vi "Build Description String.vi"(8 "error in (no error)":errorcluster, 11 "Keyboard Action in":refnum<class "Keyboard Action.lvclass">) -> (0 "error out":errorcluster, 1 "Description":string, 2 "Subtype String":string, 3 "Keyboard Action out":refnum<class "Keyboard Action.lvclass">)   [LabVIEW 2020, in "MacroAssert.lvlib" / "Keyboard Action.lvclass"]
doc: "Builds a string to describe what <B>Step</B> does."
uses:
  Keyboard Action.lvclass
  Keyboard Action.lvclass/Keyboard Action.ctl
  MacroAssert.lvlib
panel:
  in  "Virtual Key":u8(ring)=65
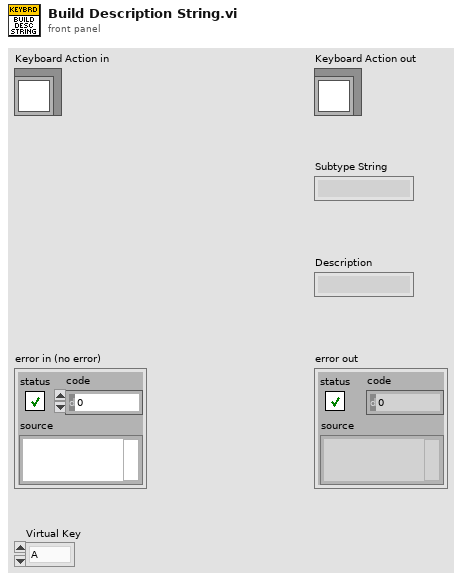
[diagram p1: front panel]
types:
  T1 = typedef "MacroAssert.lvlib/Keyboard Action.lvclass/Keyboard Action Type.ctl" = enum16{"Key Press", "Key Sequence", "Key Down", "Key Up"}
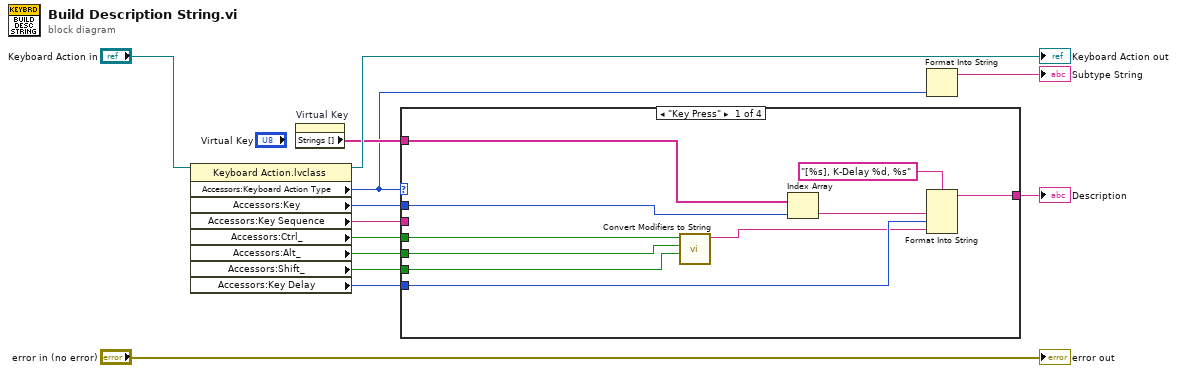
[diagram p0: block diagram]
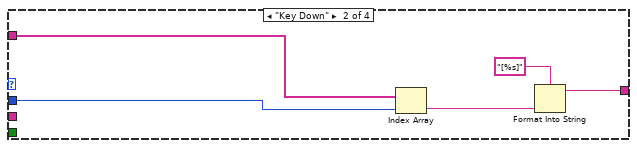
[diagram p2: hidden frame]
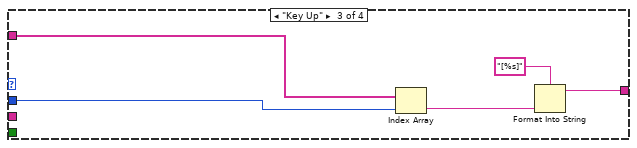
[diagram p3: hidden frame]
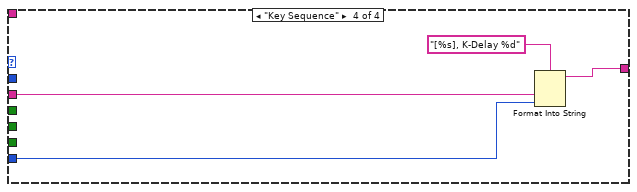
[diagram p4: hidden frame]
diagram:
  n1 = property class="Keyboard Action.lvclass"(reference="Keyboard Action in") -> (reference out=→"Keyboard Action out":refnum<class "Keyboard Action.lvclass">, "Accessors:Keyboard Action Type"=w3:T1, "Accessors:Key"=w7:u8, "Accessors:Key Sequence"=w4:string, "Accessors:Ctrl_"=w10:bool, "Accessors:Alt_"=w9:bool, "Accessors:Shift_"=w8:bool, "Accessors:Key Delay"=w6:i32)  [unwired: 1 in, 1 out]
  n2 = property on="Virtual Key" class="Ring (strict)"() -> ("Strings []"=w5:string[])  [unwired: 2 in, 2 out]
  n3 = case shown="\"Key Press\"" w3 {
    tunnel: w10 -> [w21 _ _ _]
    tunnel: w9 -> [w20 _ _ _]
    tunnel: w8 -> [w19 _ _ _]
    tunnel: w7 -> [w18 w26 w31 _]
    tunnel: [w17 w25 w30 w36] -> w1
    tunnel: w6 -> [w15 _ _ w35]
    tunnel: w5 -> [w16 w24 w29 _]
    tunnel: w4 -> [_ _ _ w34]
    frame "Key Press" {
      n4 = call "Convert Modifiers to String.vi"("Shift?"=w19, "Alt?"=w20, "Ctrl?"=w21) -> ("String"=w14:string)  [unwired: 8 in]
      n5 = Index Array(array=w16, index=w18) -> (element=w22:string)
      n6 = Format Into String(format string="[%s], K-Delay %d, %s", w22, w15, w14) -> (resulting string=w17:string)  [unwired: 2 in, 1 out]
    }
    frame "Key Down" {
      n7 = Index Array(array=w24, index=w26) -> (element=w27:string)
      n8 = Format Into String(format string="[%s]", w27) -> (resulting string=w25:string)  [unwired: 2 in, 1 out]
    }
    frame "Key Up" {
      n9 = Index Array(array=w29, index=w31) -> (element=w32:string)
      n10 = Format Into String(format string="[%s]", w32) -> (resulting string=w30:string)  [unwired: 2 in, 1 out]
    }
    frame "Key Sequence" {
      n11 = Format Into String(format string="[%s], K-Delay %d", w34, w35) -> (resulting string=w36:string)  [unwired: 2 in, 1 out]
    }
  }
  "Description" <- w1
  n12 = Format Into String(w3) -> (resulting string=→"Subtype String":string)  [unwired: 3 in, 1 out]
  "error out" <- "error in (no error)"
